vi "Read Measurement.vi"   [LabVIEW 2015, in "Agilent 2000 3000 X-Series.lvlib"]
doc: "Reads measurement results."
uses:
  <instrlib>/Agilent 2000 3000 X-Series/Agilent 2000 3000 X-Series.lvlib
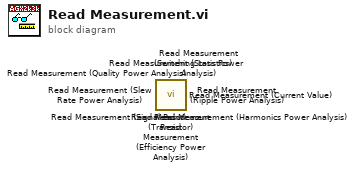
[diagram p0: block diagram]
diagram:
  n1 = call <instrlib>:"Read Measurement (Transistor).vi"() -> ()  [unwired: 13 in, 3 out]
  n2 = call <instrlib>:"Read Measurement (Switching Loss Power Analysis).vi"() -> ()  [unwired: 13 in, 3 out]
  n3 = call <instrlib>:"Read Measurement (Slew Rate Power Analysis).vi"() -> ()  [unwired: 13 in, 3 out]
  n4 = call <instrlib>:"Read Measurement (Ripple Power Analysis).vi"() -> ()  [unwired: 13 in, 3 out]
  n5 = call <instrlib>:"Read Measurement (Quality Power Analysis).vi"() -> ()  [unwired: 13 in, 3 out]
  n6 = call <instrlib>:"Read Measurement (Harmonics Power Analysis).vi"() -> ()  [unwired: 13 in, 3 out]
  n7 = call <instrlib>:"Read Measurement (Efficiency Power Analysis).vi"() -> ()  [unwired: 13 in, 3 out]
  n8 = call <instrlib>:"Read Measurement (Statistics).vi"() -> ()  [unwired: 7 in, 9 out]
  n9 = call <instrlib>:"Read Measurement (Signal Point).vi"() -> ()  [unwired: 13 in, 3 out]
  n10 = call <instrlib>:"Read Measurement (Current Value).vi"() -> ()  [unwired: 13 in, 3 out]
